vi "OneQuadProfile (SubVI).vi"(1 "corner-based \ncoordinates (pix)":dbl[](array[numeric]), 2 "Rsin(phi)[Q]":dbl[][][](array[numeric]), 3 "Rcos(phi)[Q]":dbl[][][](array[numeric]), 5 "Quadrant?":i32, 6 "Image":i32[][](array[numeric]), 7 "lengths":i32[](array[numeric])) -> (12 "profile":dbl[](array[numeric]))   [LabVIEW 2011, in "OfflineTracker.lvlib"]
uses:
  OfflineTracker.lvlib
panel:
  out "q mean":dbl
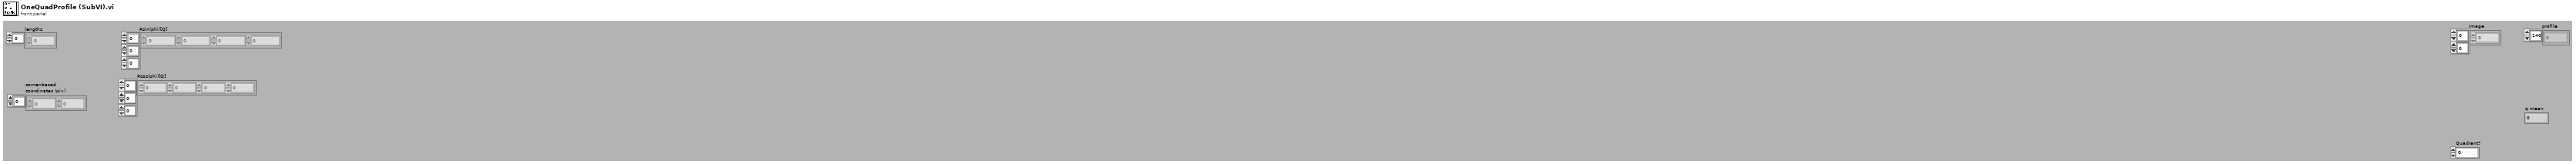
[diagram p1: front panel]
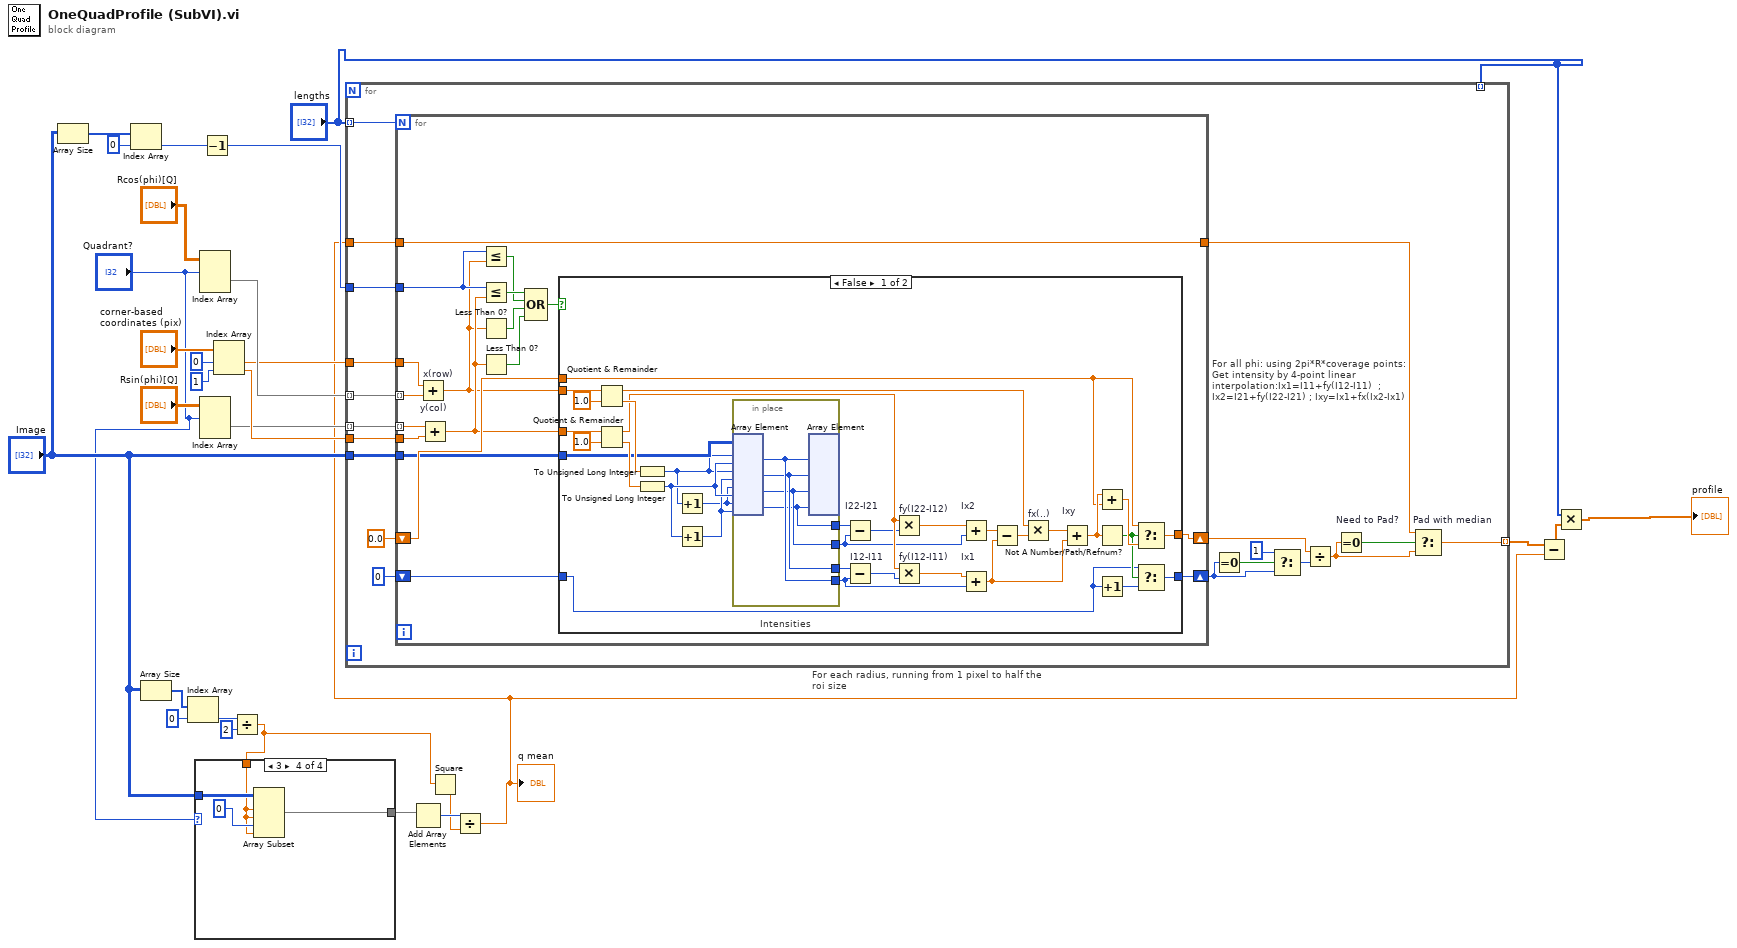
[diagram p0: block diagram]
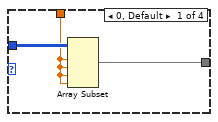
[diagram p2: hidden frame]
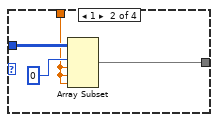
[diagram p3: hidden frame]
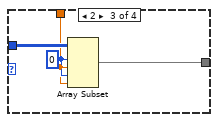
[diagram p4: hidden frame]
diagram:
  n1 = Array Size(array="Image") -> (size(s)=w19:i32[])
  n2 = Index Array(array=w19, index=0) -> (element=w17:i32)
  n3 = Array Size(array="Image") -> (size(s)=w10:i32[])
  n4 = Index Array(array=w10, index=0) -> (element=w8:i32)
  n5 = Index Array(array="Rcos(phi)[Q]", index (dim 0)="Quadrant?") -> (element=w28:dbl[][])  [unwired: 2 in]
  n6 = Index Array(array="Rsin(phi)[Q]", index (dim 0)="Quadrant?") -> (element=w20:dbl[][])  [unwired: 2 in]
  n7 = Decrement(x=w17) -> (x-1=w16:i32)
  n8 = Index Array(array="corner-based \ncoordinates (pix)", index #1=0 ("index"), index #2=1 ("index")) -> (element #1=w25:dbl, element #2=w24:dbl)
  n9 = Divide(x=w8, y=2) -> (x/y=w5:dbl)
  n10 = case shown="3" "Quadrant?" {
    tunnel: "Image" -> [w31 w35 w39 w43]
    tunnel: w5 -> [w30 w33 w37 w41]
    tunnel: [w29 w32 w36 w40] -> w3
    frame 0, Default {
      n11 = Array Subset(array=w31, index (row)=w30, length (row)=w30, index (col)=w30, length (col)=w30) -> (w29:i32[][])
    }
    frame 1 {
      n12 = Array Subset(array=w35, index (row)=0 ("index"), length (row)=w33, index (col)=w33, length (col)=w33) -> (w32:i32[][])
    }
    frame 2 {
      w38 = 0 ("index")
      n13 = Array Subset(array=w39, index (row)=w38, length (row)=w37, index (col)=w38, length (col)=w37) -> (w36:i32[][])
    }
    frame 3 {
      n14 = Array Subset(array=w43, index (row)=w41, length (row)=w41, index (col)=0 ("index"), length (col)=w41) -> (w40:i32[][])
    }
  }
  n15 = Add Array Elements(numeric array=w3) -> (sum=w4:i32)
  n16 = Square(x=w5) -> (x^2=w2:dbl)
  n17 = Divide(x=w4, y=w2) -> (x/y=w1:dbl)
  "q mean" <- w1
  n18 = for "For each radius, running from 1 pixel to half the roi size" {
    tunnel: "Image" -> [w62]
    tunnel: w25 -> [w58]
    tunnel: w24 -> [w57]
    tunnel: [w48] -> w13 mode=indexing
    tunnel: w1 -> [w45]
    tunnel: w28 -> [w51] mode=indexing
    tunnel: w20 -> [w50] mode=indexing
    tunnel: "lengths" -> [w52] mode=indexing
    tunnel: w16 -> [w47]
    tunnel: "lengths" -> [_] mode=indexing
    n19 = for "For all phi: using 2pi*R*coverage points: \nGet intensity by 4-point linear interpolation:Ix1=I11+fy(I12-I11)  ; Ix2=I21+fy(I22-I21) ; Ixy=Ix1+fx(Ix2-Ix1)" {
      N: w52 -> [_]
      tunnel: w62 -> [w77]
      shift-right: [w64] -> w60
      shift-left: 0.0 -> [w80]
      shift-right: [w65] -> w46
      shift-left: u32 0 ("milliseconds to wait") -> [w66]
      tunnel: w58 -> [w79]
      tunnel: w57 -> [w78]
      tunnel: w50 -> [w75] mode=indexing
      tunnel: w51 -> [w76] mode=indexing
      tunnel: w47 -> [w74]
      tunnel: w45 -> [w63]
      tunnel: [w63] -> w44
      n20 = Add "x(row)"(x=w79, y=w76) -> (x+y=w72:dbl)
      n21 = Add "y(col)"(x=w75, y=w78) -> (x+y=w73:dbl)
      n22 = Less Or Equal?(x=w74, y=w72) -> (x <= y?=w70:bool)
      n23 = Less Or Equal?(x=w74, y=w73) -> (x <= y?=w71:bool)
      n24 = Less Than 0?(x=w72) -> (x < 0?=w69:bool)
      n25 = Less Than 0?(x=w73) -> (x < 0?=w68:bool)
      n26 = Compound Arithmetic op=OR(w71, w70, w69, w68) -> (w67:bool)
      n27 = case shown="False" w67 {
        tunnel: w80 -> [w87 w119]
        tunnel: w73 -> [w113 _]
        tunnel: w72 -> [w112 _]
        tunnel: [w86 w119] -> w64
        tunnel: w77 -> [w105 _]
        tunnel: w66 -> [w81 w118]
        tunnel: [w83 w118] -> w65
        frame False {
          n28 = Quotient & Remainder(x=w112, y=1.0) -> (x-y*floor(x/y)=w106:dbl, floor(x/y)=w109:dbl)
          n29 = Quotient & Remainder(x=w113, y=1.0) -> (x-y*floor(x/y)=w107:dbl, floor(x/y)=w108:dbl)
          n30 = To Unsigned Long Integer(number=w109) -> (unsigned 32bit integer=w94:u32)
          n31 = To Unsigned Long Integer(number=w108) -> (unsigned 32bit integer=w96:u32)
          n32 = Increment(x=w94) -> (x+1=w93:u32)
          n33 = Increment(x=w96) -> (x+1=w95:u32)
          n34 = in-place "Intensities" {
            in-place-border: [w117] -> w89
            in-place-border: [w116] -> w90
            in-place-border: [w115] -> w91
            in-place-border: [w114] -> w92
            n35 = in-place-array #1(w105, w94, w96, w94, w95, w93, w96, w93, w95) -> (w117:i32, w116:i32, w115:i32, w114:i32)
            n36 = in-place-array #1(w117, w116, w115, w114) -> ()  [unwired: 9 out]
          }
          n37 = Subtract "I22-I21"(x=w92, y=w91) -> (x-y=w102:i32)
          n38 = Subtract "I12-I11"(x=w90, y=w89) -> (x-y=w104:i32)
          n39 = Multiply "fy(I22-I12)"(x=w107, y=w102) -> (x*y=w101:dbl)
          n40 = Multiply "fy(I12-I11)"(x=w107, y=w104) -> (x*y=w103:dbl)
          n41 = Add "Ix2"(x=w101, y=w91) -> (x+y=w98:dbl)
          n42 = Add "Ix1"(x=w103, y=w89) -> (x+y=w97:dbl)
          n43 = Subtract(x=w98, y=w97) -> (x-y=w100:dbl)
          n44 = Multiply "fx(..)"(x=w106, y=w100) -> (x*y=w99:dbl)
          n45 = Add "Ixy"(x=w99, y=w97) -> (x+y=w88:dbl)
          n46 = Add(x=w88, y=w87) -> (x+y=w85:dbl)
          n47 = Not A Number/Path/Refnum?(number/path/refnum=w88) -> (NaN/Path/Refnum?=w82:bool)
          n48 = Increment(x=w81) -> (x+1=w84:u32)
          n49 = Select(t=w87, s=w82, f=w85) -> (s? t:f=w86:dbl)
          n50 = Select(t=w81, s=w82, f=w84) -> (s? t:f=w83:u32)
        }
        frame True {
        }
      }
    }
    n51 = Equal To 0?(x=w46) -> (x = 0?=w55:bool)
    n52 = Select(t=u32 1, s=w55, f=w46) -> (s? t:f=w54:u32)
    n53 = Divide(x=w60, y=w54) -> (x/y=w49:dbl)
    n54 = Equal To 0? "Need to Pad?"(x=w49) -> (x = 0?=w53:bool)
    n55 = Select "Pad with median"(t=w44, s=w53, f=w49) -> (s? t:f=w48:dbl)
  }
  n56 = Subtract(x=w13, y=w1) -> (x-y=w15:dbl[])
  n57 = Multiply(x="lengths", y=w15) -> (x*y=→"profile":dbl[])
